vi "Login.vi"() -> ()   [LabVIEW 2017]
doc: "SubVI criada para realizar login de usuários"
uses:
  controls/Table.ctl
  controls/DataIn.ctl
  controls/Tabuleiro.ctl
  controls/GameOption.ctl
  controls/Login - States.ctl
  <vilib>/Utility/file.llb/Read Delimited Spreadsheet (string).vi
  <vilib>/Utility/file.llb/Write Delimited Spreadsheet (string).vi
panel:
  out "DataOut":T1
  in  "logout":bool
  out "Table":T4
  in  "Login":bool
  in  "User Name":string
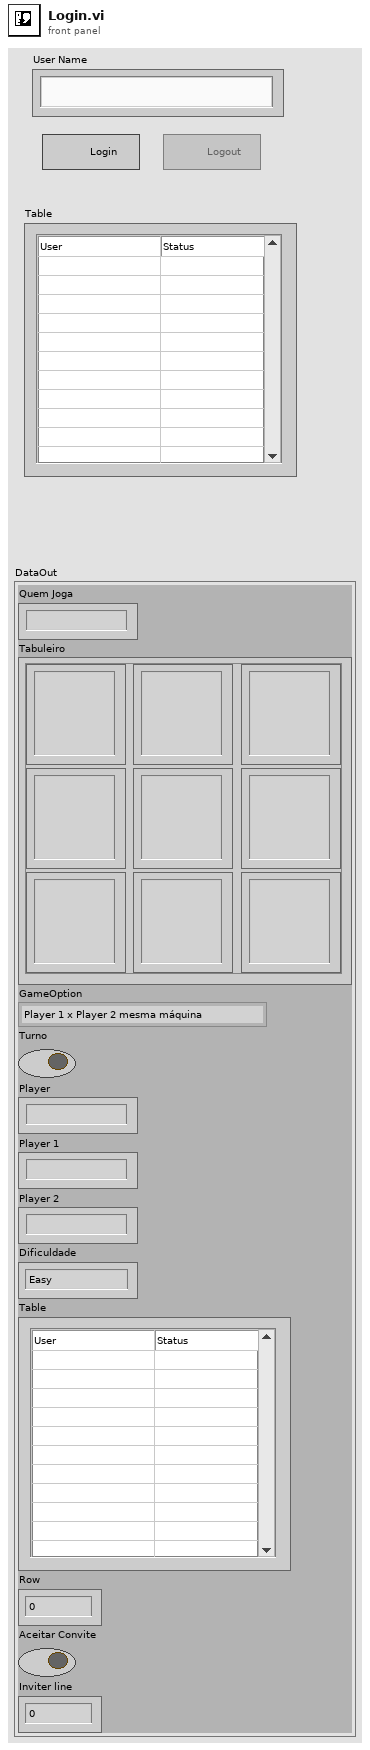
[diagram p1: front panel]
types:
  T1 = typedef "DataIn.ctl" = cluster{"Quem Joga":string, "Tabuleiro":T2, "GameOption":T3, "Turno":bool, "Player":string, "Player 1":string, "Player 2":string, "Dificuldade":enum16{"Easy", "Medium", "Hard"}, "Table":T4, "Row":u32, "Aceitar Convite":bool, "Inviter line":u32}
  T2 = typedef "Tabuleiro.ctl" = cluster{"(0,0)":string, "(1,0)":string, "(0,1)":string, "(1,1)":string, "(2,0)":string, "(1,2)":string, "(2,2)":string, "(0,2)":string, "(2,1) ":string}
  T3 = typedef "GameOption.ctl" = enum16{"Player 1 x Player 2 mesma máquina", "Player 1 x Player 2 pela rede", "Player 1 x Computador", "Wait for Event", "Initialize", "Stop"}
  T4 = typedef "Table.ctl" = string[][]
  T5 = typedef "Login - States.ctl" = enum16{"Login - Initialize", "Login - Wait for Event", "Login", "Logout", "Logout - Panel Close", "Table Refresh", "Invitation"}
  T6 = enum8{"Enabled", "Disabled", "Disabled and Grayed Out"}
  T7 = typedef "LVRowAndColumnTypeDef.ctl" = cluster{"Row":i32, "Column":i32}
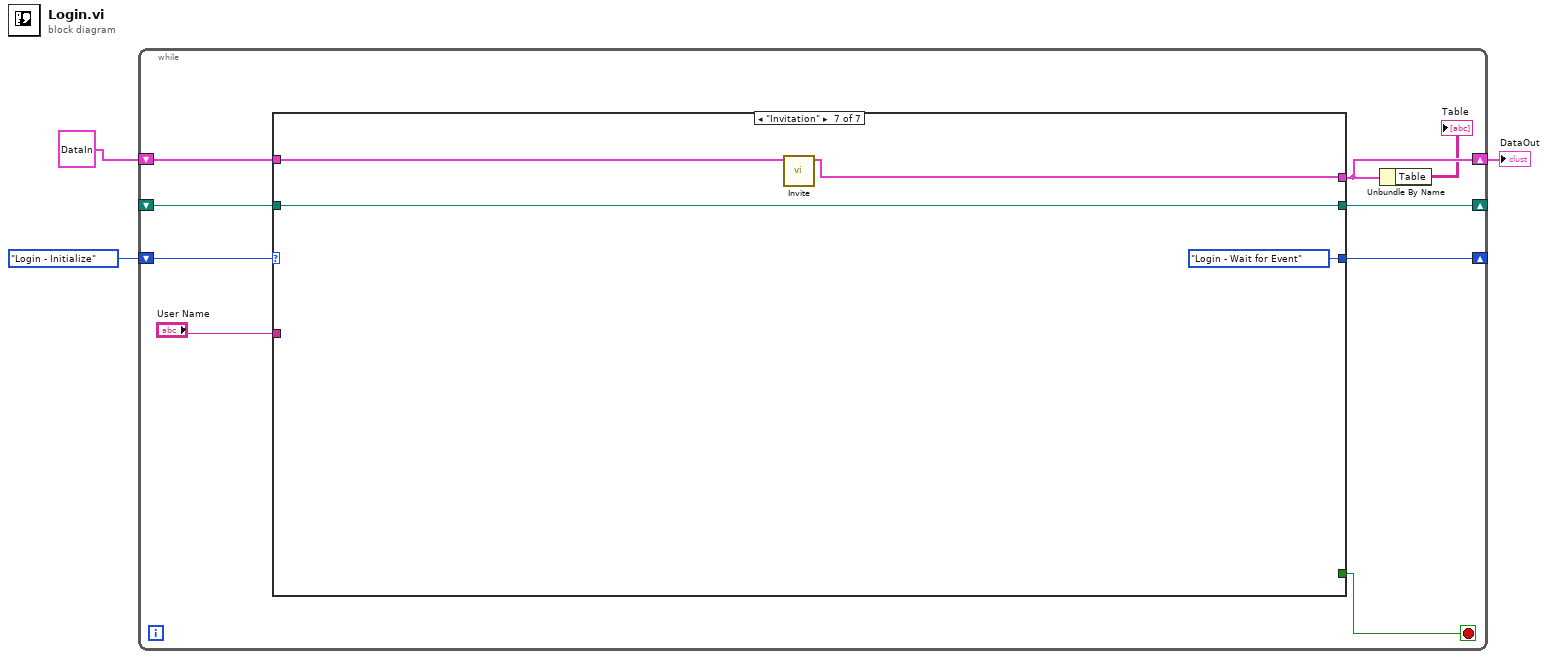
[diagram p0: block diagram]
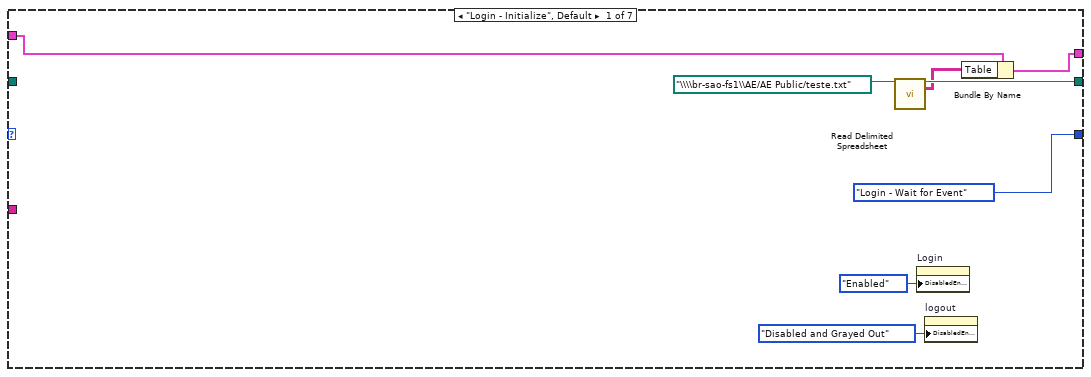
[diagram p2: hidden frame]
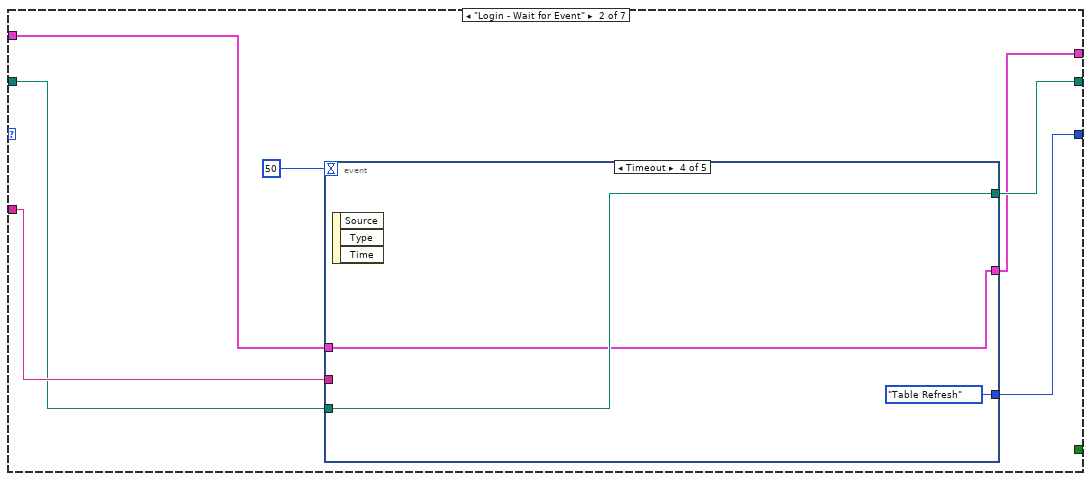
[diagram p3: hidden frame]
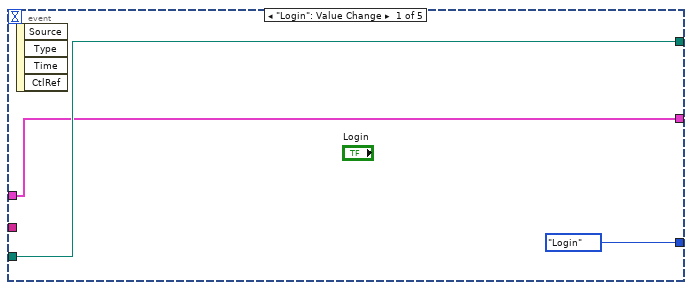
[diagram p4: hidden frame]
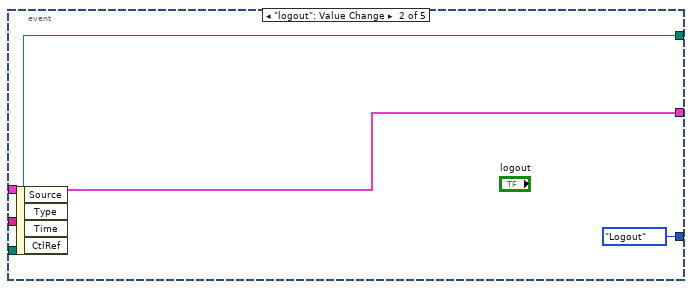
[diagram p5: hidden frame]
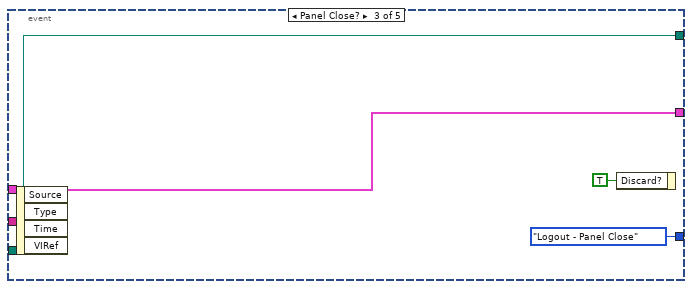
[diagram p6: hidden frame]
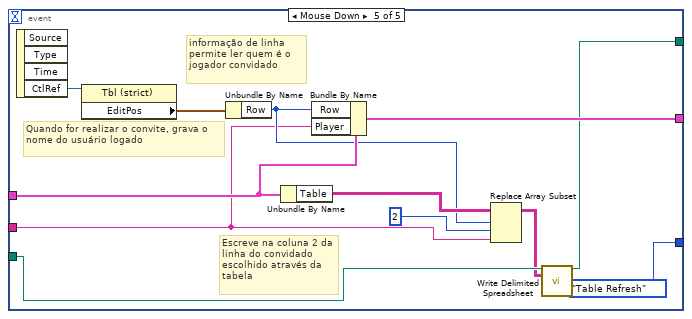
[diagram p7: hidden frame]
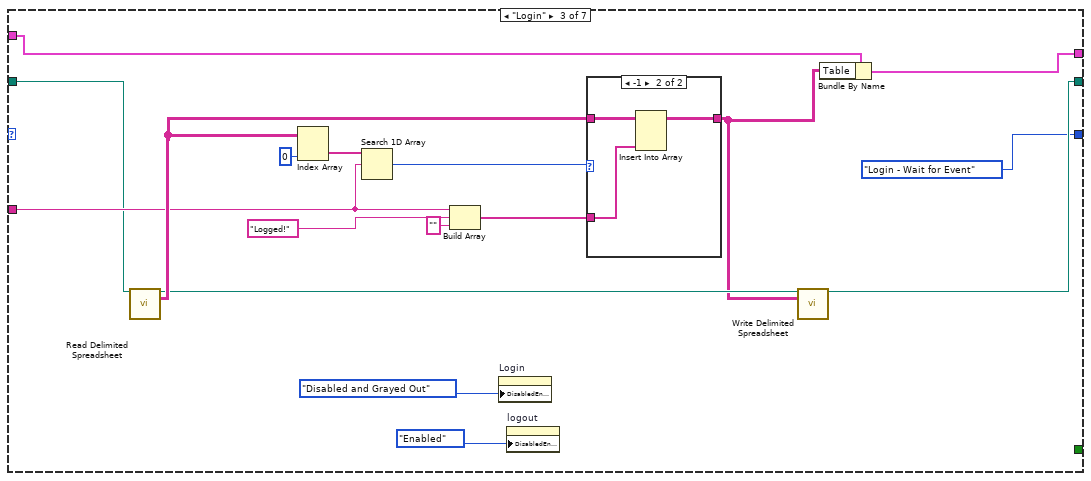
[diagram p8: hidden frame]
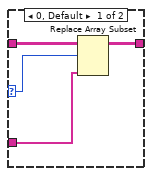
[diagram p9: hidden frame]
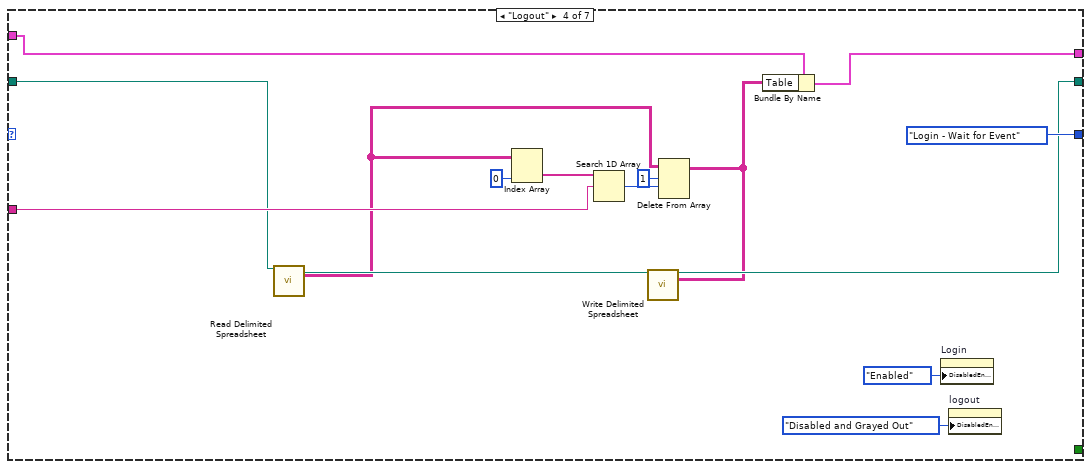
[diagram p10: hidden frame]
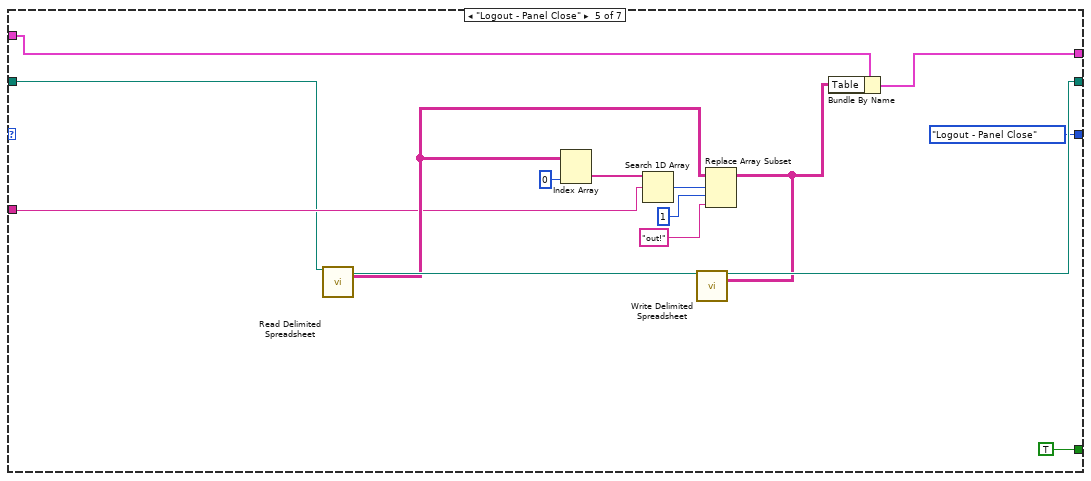
[diagram p11: hidden frame]
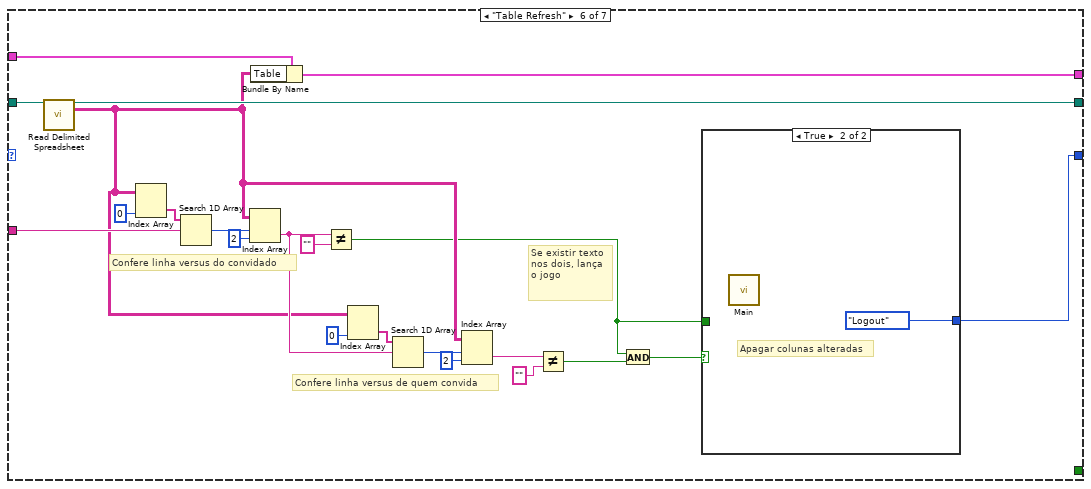
[diagram p12: hidden frame]
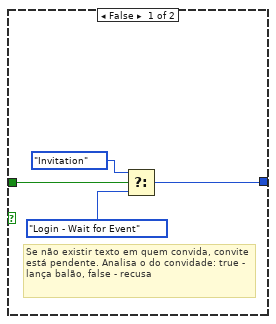
[diagram p13: hidden frame]
diagram:
  n1 = while {
    shift-right: [w11] -> _
    shift-left: Login_-_States."Login - Initialize" -> [w12]
    shift-right: [w10] -> _
    shift-left: _ -> [w9]
    shift-right: [w5] -> w1
    shift-left: T1 {"Quem Joga"="", "Tabuleiro"={"(0,0)"="", "(1,0)"="", "(0,1)"="", "(1,1)"="", "(2,0)"="", "(1,2)"="", "(2,2)"="", "(0,2)"="", "(2,1) "=""}, "GameOption"=enum."Player 1 x Player 2 mesma máquina", "Turno"=FALSE, "Player"="", "Player 1"="", "Player 2"="", "Dificuldade"=enum."Easy", "Table"=[], "Row"=0, "Aceitar Convite"=FALSE, "Inviter line"=0} ("DataIn") -> [w8]
    stop <- w6 stop-if-true
    n2 = case shown="\"Invitation\"" w12 {
      tunnel: [Login_-_States."Login - Wait for Event" w27 Login_-_States."Login - Wait for Event" Login_-_States."Login - Wait for Event" Login_-_States."Logout - Panel Close" w107 Login_-_States."Login - Wait for Event"] -> w11
      tunnel: [w18 w23 w61 w86 w98 w127 w136] -> w10
      tunnel: w9 -> [_ w24 w59 w85 w95 w128 w136]
      tunnel: w8 -> [w15 w22 w55 w79 w94 w120 w135]
      tunnel: "User Name" -> [_ w25 w62 w88 w99 w124 _]
      tunnel: [_ _ _ _ TRUE _ _] -> w6
      tunnel: [w14 w21 w54 w78 w93 w119 w134] -> w5
      frame "Login - Initialize", Default {
        n3 = call-poly <vilib>:"Read Delimited Spreadsheet.vi"("file path (dialog if empty)"=path "\\\\br-sao-fs1\\AE/AE Public/teste.txt" ("file path (use dialog)")) -> ("new file path (Not A Path if cancelled)"=w18:path, "all rows"=w13:string[][])  [unwired: 9 in, 4 out]
        n4 = property on="Login" class="Bool"("DisabledEnum"=T6."Enabled" ("Disabled")) -> ()  [unwired: 2 in, 2 out]
        n5 = property on="logout" class="Bool"("DisabledEnum"=T6."Disabled and Grayed Out" ("Disabled")) -> ()  [unwired: 2 in, 2 out]
        n6 = Bundle By Name(cluster=w15, "Table"=w13) -> (w14:T1)
      }
      frame "Login - Wait for Event" {
        n7 = event shown="[3] Timeout" {
          selector: _ -> [_ _ _ _ _]
          dyn-events: _ -> [_ _ _ _ _]
          timeout: 50 -> [_ _ _ _ _]
          tunnel: [Login_-_States."Login" Login_-_States."Logout" Login_-_States."Logout - Panel Close" Login_-_States."Table Refresh" Login_-_States."Table Refresh"] -> w27
          tunnel: w22 -> [w28 w31 w34 w38 w46]
          tunnel: [w28 w31 w34 w38 w49] -> w21
          tunnel: w25 -> [_ _ _ _ w41]
          tunnel: w24 -> [w29 w32 w35 w39 w48]
          tunnel: [w29 w32 w35 w39 w47] -> w23
          event "Login": Value Change {
            n8 = event-data() -> ()  [unwired: 1 in, 4 out]
          }
          event "logout": Value Change {
            n9 = event-data() -> ()  [unwired: 1 in, 4 out]
          }
          event Panel Close? {
            n10 = event-data() -> ()  [unwired: 1 in, 4 out]
            n11 = event-data("Discard?"=TRUE) -> ()  [unwired: 1 in, 1 out]
          }
          event Timeout {
            n12 = event-data() -> ()  [unwired: 1 in, 3 out]
          }
          event Mouse Down {
            # "Escreve na coluna 2 da linha do convidado escolhido através da tabela"
            # "Quando for realizar o convite, grava o nome do usuário logado"
            # "informação de linha permite ler quem é o jogador convidado"
            n13 = event-data() -> ("CtlRef"=w51:refnum<vi>)  [unwired: 1 in, 3 out]
            n14 = property class="Tbl (strict)"(reference=w51) -> ("EditPos"=w50:T7)  [unwired: 1 in, 2 out]
            n15 = Unbundle By Name(w50) -> ("Row"=w43:i32)
            n16 = Unbundle By Name(w46) -> ("Table"=w45:T4)
            n17 = Bundle By Name(cluster=w46, "Row"=w43, "Player"=w41) -> (w49:T1)
            n18 = Replace Array Subset(array=w45, new element=w41, index (row)=w43, index (col)=2 ("disabled index (col)")) -> (w44:T4)
            n19 = call-poly <vilib>:"Write Delimited Spreadsheet.vi"("file path (dialog if empty)"=w48, "2D data"=w44) -> ("new file path (Not A Path if cancelled)"=w47:path)  [unwired: 12 in, 1 out]
          }
        }
      }
      frame "Login" {
        n20 = call-poly <vilib>:"Read Delimited Spreadsheet.vi"("file path (dialog if empty)"=w59) -> ("new file path (Not A Path if cancelled)"=w68:path, "all rows"=w69:string[][])  [unwired: 9 in, 4 out]
        n21 = Index Array(array=w69, index (col)=0 ("index (row)")) -> (element=w63:string[])  [unwired: 1 in]
        n22 = Search 1D Array(1D array=w63, element=w62) -> (index of element=w67:i32)  [unwired: 1 in]
        n23 = Build Array(w62, "Logged!" ("input 2"), "" ("element")) -> (w65:string[])
        n24 = property on="Login" class="Bool"("DisabledEnum"=T6."Disabled and Grayed Out" ("Disabled")) -> ()  [unwired: 2 in, 2 out]
        n25 = property on="logout" class="Bool"("DisabledEnum"=T6."Enabled" ("Disabled")) -> ()  [unwired: 2 in, 2 out]
        n26 = case shown="-1" w67 {
          selector: w67 -> [w70 _]
          tunnel: w69 -> [w73 w76]
          tunnel: w65 -> [w72 w75]
          tunnel: [w71 w74] -> w53
          frame 0, Default {
            n27 = Replace Array Subset(array=w73, new element=w72, index (row)=w70) -> (w71:string[][])  [unwired: 1 in]
          }
          frame -1 {
            n28 = Insert Into Array(array=w76, new element=w75) -> (w74:string[][])  [unwired: 2 in]
          }
        }
        n29 = call-poly <vilib>:"Write Delimited Spreadsheet.vi"("file path (dialog if empty)"=w68, "2D data"=w53) -> ("new file path (Not A Path if cancelled)"=w61:path)  [unwired: 12 in, 1 out]
        n30 = Bundle By Name(cluster=w55, "Table"=w53) -> (w54:T1)
      }
      frame "Logout" {
        n31 = call-poly <vilib>:"Read Delimited Spreadsheet.vi"("file path (dialog if empty)"=w85) -> ("new file path (Not A Path if cancelled)"=w91:path, "all rows"=w82:string[][])  [unwired: 9 in, 4 out]
        n32 = Index Array(array=w82, index (col)=0 ("disabled index (col)")) -> (element=w90:string[])  [unwired: 1 in]
        n33 = Search 1D Array(1D array=w90, element=w88) -> (index of element=w81:i32)  [unwired: 1 in]
        n34 = Delete From Array(array=w82, length=1, index (row)=w81) -> (array with subset deleted=w77:string[][])  [unwired: 1 in, 1 out]
        n35 = call-poly <vilib>:"Write Delimited Spreadsheet.vi"("file path (dialog if empty)"=w91, "2D data"=w77) -> ("new file path (Not A Path if cancelled)"=w86:path)  [unwired: 12 in, 1 out]
        n36 = Bundle By Name(cluster=w79, "Table"=w77) -> (w78:T1)
        n37 = property on="Login" class="Bool"("DisabledEnum"=T6."Enabled" ("Disabled")) -> ()  [unwired: 2 in, 2 out]
        n38 = property on="logout" class="Bool"("DisabledEnum"=T6."Disabled and Grayed Out" ("Disabled")) -> ()  [unwired: 2 in, 2 out]
      }
      frame "Logout - Panel Close" {
        n39 = call-poly <vilib>:"Read Delimited Spreadsheet.vi"("file path (dialog if empty)"=w95) -> ("new file path (Not A Path if cancelled)"=w106:path, "all rows"=w104:string[][])  [unwired: 9 in, 4 out]
        n40 = Index Array(array=w104, index (col)=0 ("disabled index (col)")) -> (element=w103:string[])  [unwired: 1 in]
        n41 = Search 1D Array(1D array=w103, element=w99) -> (index of element=w105:i32)  [unwired: 1 in]
        n42 = Replace Array Subset(array=w104, new element="out!" ("element"), index (row)=w105, index (col)=1 ("disabled index (col)")) -> (w92:string[][])
        n43 = call-poly <vilib>:"Write Delimited Spreadsheet.vi"("file path (dialog if empty)"=w106, "2D data"=w92) -> ("new file path (Not A Path if cancelled)"=w98:path)  [unwired: 12 in, 1 out]
        n44 = Bundle By Name(cluster=w94, "Table"=w92) -> (w93:T1)
      }
      frame "Table Refresh" {
        # "Se existir texto nos dois, lança o jogo"
        # "Confere linha versus de quem convida"
        # "Confere linha versus do convidado"
        n45 = call-poly <vilib>:"Read Delimited Spreadsheet.vi"("file path (dialog if empty)"=w128) -> ("new file path (Not A Path if cancelled)"=w127:path, "all rows"=w112:string[][])  [unwired: 9 in, 4 out]
        n46 = Index Array(array=w112, index (col)=0 ("disabled index (col)")) -> (element=w125:string[])  [unwired: 1 in]
        n47 = Search 1D Array(1D array=w125, element=w124) -> (index of element=w121:i32)  [unwired: 1 in]
        n48 = Index Array(array=w112, index (row)=w121, index (col)=2) -> (element=w113:string)
        n49 = Bundle By Name(cluster=w120, "Table"=w112) -> (w119:T1)
        n50 = Not Equal?(x=w113, y="") -> (x != y?=w108:bool)
        n51 = Index Array(array=w112, index (col)=0 ("disabled index (col)")) -> (element=w115:string[])  [unwired: 1 in]
        n52 = Search 1D Array(1D array=w115, element=w113) -> (index of element=w118:i32)  [unwired: 1 in]
        n53 = Index Array(array=w112, index (row)=w118, index (col)=2) -> (element=w111:string)
        n54 = Not Equal?(x=w111, y="") -> (x != y?=w110:bool)
        n55 = And(x=w108, y=w110) -> (x .and. y?=w109:bool)
        n56 = case shown="True" w109 {
          tunnel: w108 -> [w132 _]
          tunnel: [w129 Login_-_States."Logout"] -> w107
          frame False {
            # "Se não existir texto em quem convida, convite está pendente. Analisa o do convidade: true - lança balão, false - recusa"
            n57 = Select(t=Login_-_States."Invitation" ("f"), s=w132, f=Login_-_States."Login - Wait for Event") -> (s? t:f=w129:T5)
          }
          frame True {
            # "Apagar colunas alteradas"
            n58 = call "Main.vi"() -> ()  [unwired: 11 in, 1 out]
          }
        }
      }
      frame "Invitation" {
        n59 = call "Invite.vi"("DataIn"=w135) -> ("DataOut"=w134:T1)  [unwired: 9 in]
      }
    }
    n60 = Unbundle By Name(w5) -> ("Table"=→"Table":T4)
  }
  "DataOut" <- w1
